vi "tankdrive printout.vi"() -> ()   [LabVIEW 2012, in "Omni2013.lvrbt"]
uses:
  Omni2013.lvrbt
  <vilib>/NXT/Dual Mode Library/Logging/CreateLoggingFile.vi
  <vilib>/FTC/FTC Calculate Drive Power - Arcade Left.vi
  <vilib>/NXT/Dual Mode Library/Display/drawNumber.vi
  <vilib>/NXT/Dual Mode Library/Display/drawText_Center.vi
panel:
  in  "Drive Power":i8=100 min=-100 max=100
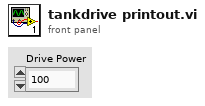
[diagram p1: front panel]
types:
  T1 = typedef "LVHSConnector.ctl" = refnum<class "BrickReference.lvclass">
  T2 = typedef "FTC ControllerState.ctl" = cluster{"Left X":i8, "Left Y":i8, "Right X":i8, "Right Y":i8, "Button Encoding 9-12":u8, "Button Encoding 1-8":u8, "POV":T3}
  T3 = typedef "FTC POVState.ctl" = i8
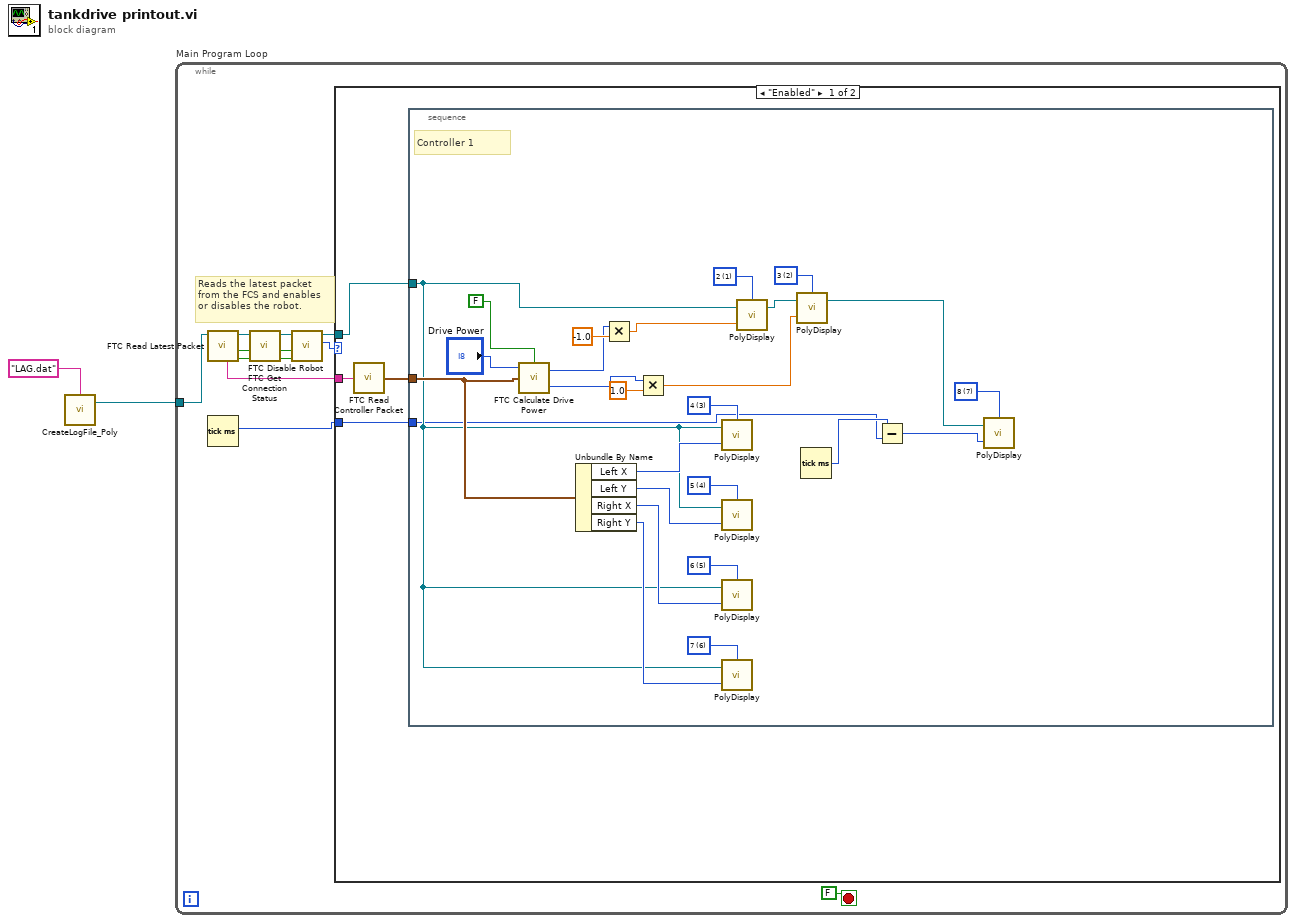
[diagram p0: block diagram]
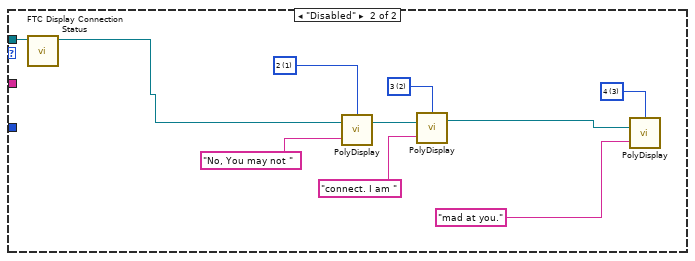
[diagram p2: hidden frame]
diagram:
  n1 = call-poly <vilib>:"CreateLogFile_Poly.vi"("Filename"="LAG.dat") -> ("NXT"=w1:T1)  [unwired: 3 in]
  n2 = while "Main Program Loop" {
    tunnel: w1 -> [w3]
    stop <- FALSE stop-if-true
    # "Reads the latest packet\nfrom the FCS and enables\nor disables the robot."
    n3 = call <vilib>:"FTC Read Latest Packet.vi"("NXT"=w3) -> ("Packet Received?"=w12:bool, "Stopped?"=w9:bool, "NXT"=w11:T1, "Controller 1"=w13:string)  [unwired: 5 in, 2 out]
    n4 = Tick Count (ms)() -> (millisecond timer value=w4:u32)
    n5 = call <vilib>:"FTC Get Connection Status.vi"("Packet Received?"=w12, "Stopped?"=w9, "NXT"=w11) -> ("Online?"=w6:bool, "Stopped?"=w7:bool, "NXT"=w8:T1)  [unwired: 5 in]
    n6 = call <vilib>:"FTC Disable Robot.vi"("Online?"=w6, "Stopped?"=w7, "NXT"=w8) -> ("Enabled?"=w10:enum16{"Disabled", "Enabled"}, "NXT"=w5:T1)  [unwired: 3 in]
    n7 = case "disableCase" shown="\"Enabled\"" w10 {
      tunnel: w13 -> [w18 _]
      tunnel: w5 -> [w16 w54]
      tunnel: w4 -> [w15 _]
      frame "Enabled" {
        n8 = call <vilib>:"FTC Read Controller Packet.vi"("Packet"=w18) -> ("Controller State"=w17:T2)  [unwired: 4 in]
        n9 = stacked-sequence "controller1Actions" {
          tunnel: w17 -> [w33]
          tunnel: w16 -> [w24]
          tunnel: w15 -> [w19]
          frame #0 {
            w23 = i16 7 items=["1", "2", "3", "4", "5", "6", "7", "8"] ("Line")
            w25 = i16 6 items=["1", "2", "3", "4", "5", "6", "7", "8"] ("Line")
            w26 = i16 5 items=["1", "2", "3", "4", "5", "6", "7", "8"] ("Line")
            w27 = i16 4 items=["1", "2", "3", "4", "5", "6", "7", "8"] ("Line")
            w28 = i16 3 items=["1", "2", "3", "4", "5", "6", "7", "8"] ("Line")
            w41 = i16 2 items=["1", "2", "3", "4", "5", "6", "7", "8"] ("Line")
            w42 = i16 1 items=["1", "2", "3", "4", "5", "6", "7", "8"] ("Line")
            # "Controller 1"
            n10 = call-poly <vilib>:"FTC Calculate Drive Power.vi"("Reverse"=FALSE, "Controller State"=w33, "Power Level (50)"="Drive Power") -> ("Right Motor Power"=w37:i8, "Left Motor Power"=w38:i8)  [unwired: 1 in]
            n11 = Unbundle By Name(w33) -> ("Left X"=w32:i8, "Left Y"=w31:i8, "Right X"=w30:i8, "Right Y"=w29:i8)
            n12 = Multiply(x=w38, y=-1.0) -> (x*y=w34:dbl)
            n13 = Multiply(x=w37, y=1.0) -> (x*y=w35:dbl)
            n14 = call-poly <vilib>:"PolyDisplay.vi"("number"=w32, "NXT"=w24, "Line"=w28) -> ()  [unwired: 1 in, 1 out]
            n15 = call-poly <vilib>:"PolyDisplay.vi"("number"=w31, "NXT"=w24, "Line"=w27) -> ()  [unwired: 1 in, 1 out]
            n16 = call-poly <vilib>:"PolyDisplay.vi"("number"=w30, "NXT"=w24, "Line"=w26) -> ()  [unwired: 1 in, 1 out]
            n17 = call-poly <vilib>:"PolyDisplay.vi"("number"=w29, "NXT"=w24, "Line"=w25) -> ()  [unwired: 1 in, 1 out]
            n18 = call-poly <vilib>:"PolyDisplay.vi"("number"=w34, "NXT"=w24, "Line"=w42) -> ("NXT"=w36:T1)  [unwired: 1 in]
            n19 = call-poly <vilib>:"PolyDisplay.vi"("number"=w35, "NXT"=w36, "Line"=w41) -> ("NXT"=w21:T1)  [unwired: 1 in]
            n20 = Tick Count (ms)() -> (millisecond timer value=w20:u32)
            n21 = Subtract(x=w20, y=w19) -> (x-y=w22:u32)
            n22 = call-poly <vilib>:"PolyDisplay.vi"("number"=w22, "NXT"=w21, "Line"=w23) -> ()  [unwired: 1 in, 1 out]
          }
        }
      }
      frame "Disabled" {
        w48 = i16 3 items=["1", "2", "3", "4", "5", "6", "7", "8"] ("Line")
        w53 = i16 2 items=["1", "2", "3", "4", "5", "6", "7", "8"] ("Line")
        w49 = i16 1 items=["1", "2", "3", "4", "5", "6", "7", "8"] ("Line")
        n23 = call <vilib>:"FTC Display Connection Status.vi"("NXT"=w54) -> ("NXT"=w45:T1)  [unwired: 10 in]
        n24 = call-poly <vilib>:"PolyDisplay.vi"("Text"="No, You may not ", "NXT"=w45, "Line"=w49) -> ("NXT"=w51:T1)  [unwired: 1 in]
        n25 = call-poly <vilib>:"PolyDisplay.vi"("Text"="connect. I am ", "NXT"=w51, "Line"=w53) -> ("NXT"=w47:T1)  [unwired: 1 in]
        n26 = call-poly <vilib>:"PolyDisplay.vi"("Text"="mad at you.", "NXT"=w47, "Line"=w48) -> ()  [unwired: 1 in, 1 out]
      }
    }
  }
